vi "Getlimit.vi"(8 "error in (no error)":errorcluster, 11 "B&K Precision 9120 series in":refnum<class "B&K Precision 9120 series.lvclass">) -> (0 "error out":errorcluster, 1 "Current read":dbl, 2 "Voltage read":dbl, 3 "B&K Precision 9120 series out":refnum<class "B&K Precision 9120 series.lvclass">)   [LabVIEW 2014, in "B&K Precision 9120 series.lvclass"]
uses:
  B&K Precision 9120 series.lvclass
  B&K Precision 9120 series.lvclass/B&K Precision 9120 series.ctl
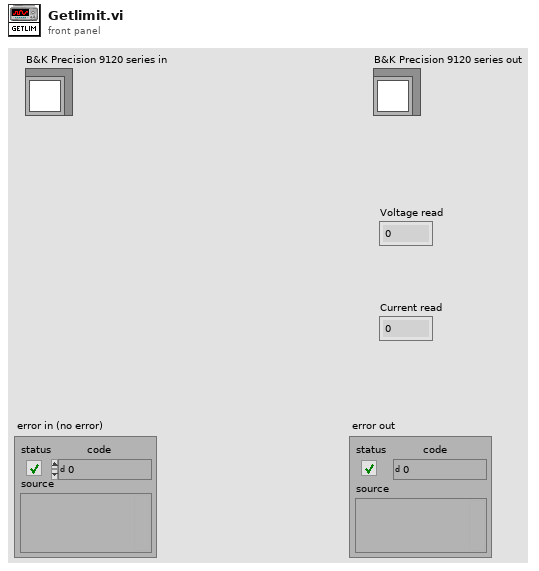
[diagram p1: front panel]
types:
  T1 = typedef "B&K Precision 9120 series.lvclass/Serial_Config.ctl" = cluster{"Baud":u32, "Flow Ctl":u16, "COM port":refnum<visa-resource-name>, "Parity":u16}
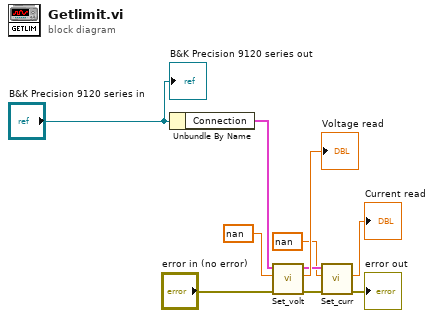
[diagram p0: block diagram]
diagram:
  n1 = Unbundle By Name("B&K Precision 9120 series in") -> ("Connection"=w10:T1)
  n2 = call "Set_volt.vi"("error in (no error)"="error in (no error)", "Voltage"=nan, "Connection in"=w10) -> ("error out"=w2:errorcluster, "actual voltage"=→"Voltage read":dbl, "Connection out"=w7:T1)  [unwired: 6 in]
  n3 = call "Set_curr.vi"("error in (no error)"=w2, "Current"=nan, "Connection in"=w7) -> ("error out"=→"error out":errorcluster, "actual current"=→"Current read":dbl)  [unwired: 6 in, 1 out]
  "B&K Precision 9120 series out" <- "B&K Precision 9120 series in"
